vi "ADDIS_detection.vi"() -> ()   [LabVIEW 2011]
panel:
  out "String (OCR/OCV 1)":string
  out "Number of Matches (Pattern Matching 1)":i32
  out "Image Out 2":T1(plugin-control)
  in  "Stop (F)":bool
  out "Image Out":T1(plugin-control)
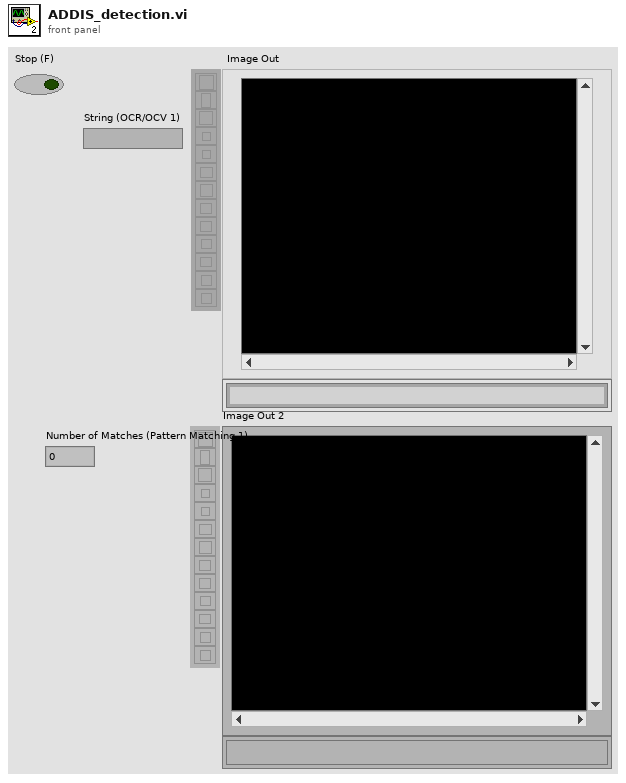
[diagram p1: front panel]
types:
  T1 = typedef "IMAQ Image.ctl" = refnum<image>
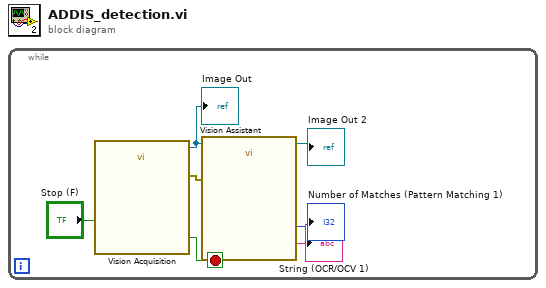
[diagram p0: block diagram]
diagram:
  n1 = while {
    stop <- w6 stop-if-true
    n2 = call "Vision Acquisition"("Stop (F)"="Stop (F)") -> ("Image Out"=w5:T1, "Stopped"=w6:bool, "error out"=w4:errorcluster)  [unwired: 24 in]
    "Image Out" <- w5
    n3 = call "Vision Assistant"("Image In"=w5, "error in"=w4) -> ("Image Out"=→"Image Out 2":T1, "Number of Matches (Pattern Matching 1)"=→"Number of Matches (Pattern Matching 1)":i32, "String (OCR/OCV 1)"=→"String (OCR/OCV 1)":string)  [unwired: 21 in, 2 out]
  }
